vi "SW_Save_parameter_group.vi"(7 "Settings file refnum in":T1, 8 "error in":errorcluster, 9 "Parameter value":string, 10 "Param group":string, 11 "Researcher name":string) -> (0 "error out":errorcluster, 2 "found?":bool, 3 "Settings file refnum out":T1)   [LabVIEW 2018]
uses:
  <vilib>/Utility/config.llb/Config Data RefNum.ctl
  <vilib>/Utility/config.llb/Write Key (String).vi
  <vilib>/Utility/config.llb/NI_LVConfig.lvlib
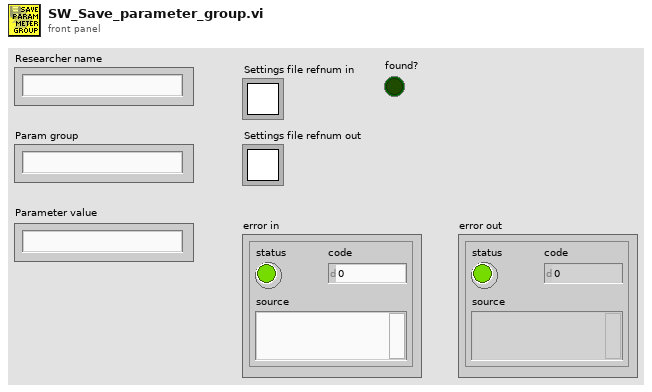
[diagram p1: front panel]
types:
  T1 = typedef "NI_LVConfig.lvlib/Config Data RefNum.ctl" = refnum<k1>
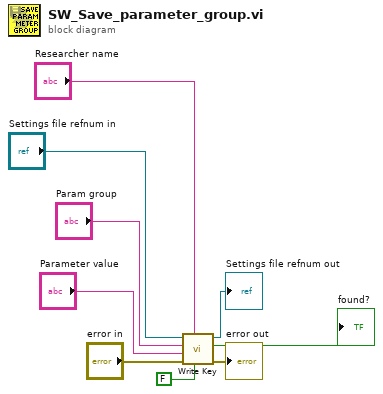
[diagram p0: block diagram]
diagram:
  n1 = call-poly <vilib>:"Write Key.vi"("write raw string? (F)"=FALSE ("read raw string? (F)"), "section"="Researcher name", "error in (no error)"="error in", "value"="Parameter value", "key"="Param group", "refnum"="Settings file refnum in") -> ("error out"=→"error out":errorcluster, "found?"=→"found?":bool, "refnum out"=→"Settings file refnum out":T1)  [unwired: 3 in]
